vi "Init Robot - Copy.vi"(8 "Brake Switch 35":bool=TRUE, 9 "Brake Switch 40":bool=TRUE, 10 "Brake 40":bool=TRUE, 11 "Brake 35":bool=TRUE) -> (0 "Force bias PS_R":dbl, 1 "Force bias GR_R":dbl, 2 "Potentiometers Diff Too Much":bool, 3 "Init values":dbl[](array[numeric]), 4 "Force Sensor Faulty":bool, 5 "Bias PS_L":dbl, 7 "Bias GR_L":dbl)   [LabVIEW 2019]
uses:
  <vilib>/myRIO/Common/Instrument Driver Framework/myRIO v1.0/Encoder/typedefs/Encoder Count Direction Enum.ctl
  <vilib>/myRIO/Common/Instrument Driver Framework/myRIO v1.0/Encoder/typedefs/Encoder Signal Mode.ctl
  <vilib>/myRIO/Common/Instrument Driver Framework/myRIO v1.0/Encoder/typedefs/Encoder Channels Enum.ctl
  <vilib>/myRIO/Common/Instrument Driver Framework/Utilities/typedefs/Generic FPGA Reference.ctl
  <vilib>/myRIO/Common/Instrument Driver Framework/Utilities/typedefs/myRIO v1.0 Reference.ctl
  <vilib>/myRIO/Common/Instrument Driver Framework/Utilities/typedefs/Hardware Version Enum.ctl
  <vilib>/myRIO/Common/Instrument Driver Framework/Utilities/typedefs/myRIO Generic Hardware Reference.ctl
  <vilib>/myRIO/Instrument Drivers/Onboard IO/Encoder/typedefs/Encoder Reference.ctl
  <vilib>/myRIO/Instrument Drivers/Onboard IO/Encoder/Encoder.lvlib
  <vilib>/myRIO/Instrument Drivers/Onboard IO/Encoder/vis/Read.vi
  <vilib>/myRIO/Common/Instrument Driver Framework/myRIO v1.0/Encoder/typedefs/Encoder Configuration v1.0.ctl
  <vilib>/userDefined/High Color/nirio_resource_hc.ctl
  <vilib>/myRIO/Common/Instrument Driver Framework/myRIO v1.0/Encoder/vis/myRIO v1.0 Configure Encoder.vi
  <vilib>/myRIO/Instrument Drivers/Onboard IO/Encoder/vis/myRIO Encoder Open.xnode
  <vilib>/myRIO/Common/Instrument Driver Framework/Utilities/vis/Is FPGA Ref Available.vi
  <vilib>/myRIO/Express VI/Onboard IO/Encoder/Encoder Express VI.xnode
  <vilib>/myRIO/Express VI/Onboard IO/DO/DO Express VI.xnode
  <vilib>/myRIO/Instrument Drivers/Onboard IO/DIO/vis/Write.vi
  <vilib>/myRIO/Instrument Drivers/Onboard IO/DIO/DIO.lvlib
  <vilib>/myRIO/Common/Instrument Driver Framework/myRIO v1.0/DIO/typedefs/DIO Channels Enum.ctl
  <vilib>/myRIO/Common/Instrument Driver Framework/myRIO v1.0/DIO/typedefs/DIO Channels List.ctl
  <vilib>/myRIO/Instrument Drivers/Onboard IO/DIO/typedefs/DIO Reference.ctl
  <vilib>/myRIO/Instrument Drivers/Onboard IO/DIO/vis/myRIO DIO Open.xnode
  <vilib>/myRIO/Express VI/Onboard IO/AI/AI Express VI.xnode
  <vilib>/myRIO/Common/Instrument Driver Framework/Utilities/typedefs/Analog Scaling Constants.ctl
  <vilib>/myRIO/Common/Instrument Driver Framework/Utilities/typedefs/Analog Scaling Constants List.ctl
  <vilib>/myRIO/Common/Instrument Driver Framework/myRIO v1.0/AO/typedefs/AO Channels Enum.ctl
  <vilib>/myRIO/Common/Instrument Driver Framework/myRIO v1.0/AO/typedefs/AO Channels List.ctl
  <vilib>/myRIO/Instrument Drivers/Onboard IO/AO/typedefs/AO Reference.ctl
  <vilib>/myRIO/Instrument Drivers/Onboard IO/AO/AO.lvlib
  <vilib>/myRIO/Instrument Drivers/Onboard IO/AO/vis/Write.vi
  <vilib>/myRIO/Instrument Drivers/Onboard IO/AO/vis/myRIO AO Open.xnode
  <vilib>/myRIO/Express VI/Onboard IO/AO/AO Express VI.xnode
  <vilib>/myRIO/Instrument Drivers/Onboard IO/AI/vis/Read.vi
  <vilib>/myRIO/Instrument Drivers/Onboard IO/AI/AI.lvlib
  <vilib>/myRIO/Common/Instrument Driver Framework/myRIO v1.0/AI/typedefs/AI Channels Enum.ctl
  <vilib>/myRIO/Common/Instrument Driver Framework/myRIO v1.0/AI/typedefs/AI Channels List.ctl
  <vilib>/myRIO/Instrument Drivers/Onboard IO/AI/typedefs/AI Reference.ctl
  <vilib>/myRIO/Instrument Drivers/Onboard IO/AI/vis/myRIO AI Open.xnode
  <vilib>/myRIO/Common/Instrument Driver Framework/myRIO v1.0/DIO/vis/myRIO v1.1 Open DIO.vi
  <vilib>/myRIO/Common/Instrument Driver Framework/myRIO v1.0/AI/vis/myRIO v1.1 Open AI.vi
  <vilib>/myRIO/Common/Instrument Driver Framework/myRIO v1.0/Encoder/vis/myRIO v1.1 Open Encoder.vi
  <vilib>/myRIO/Common/Instrument Driver Framework/myRIO v1.0/AO/vis/myRIO v1.1 Open AO.vi
panel:
  out "Init Values":dbl[](array[numeric])
  out "Bias GR_R":dbl
  out "Bias PS_R":dbl
  out "VoltageTranslation":dbl
  out "VoltageRotation":dbl
  out "Force bias PS_L":dbl
  out "Force bias GR_L":dbl
  out "Encoder Counter Value":i32(graph)
  out "Encoder Counter Value 2":i32(graph)
  out "Volt L":dbl
  out "Rot Volt":dbl
  out "Volt R":dbl
  out "E rotation":dbl
  out "E translation":dbl
  out "P Rotation":dbl
  out "P Translation":dbl
  out "left init":dbl
  out "right init":dbl
  out "SCAIME":dbl
  # "This Vi starts all task, calculates the initals values of all sensores and encoder and can open the brakes if needed."
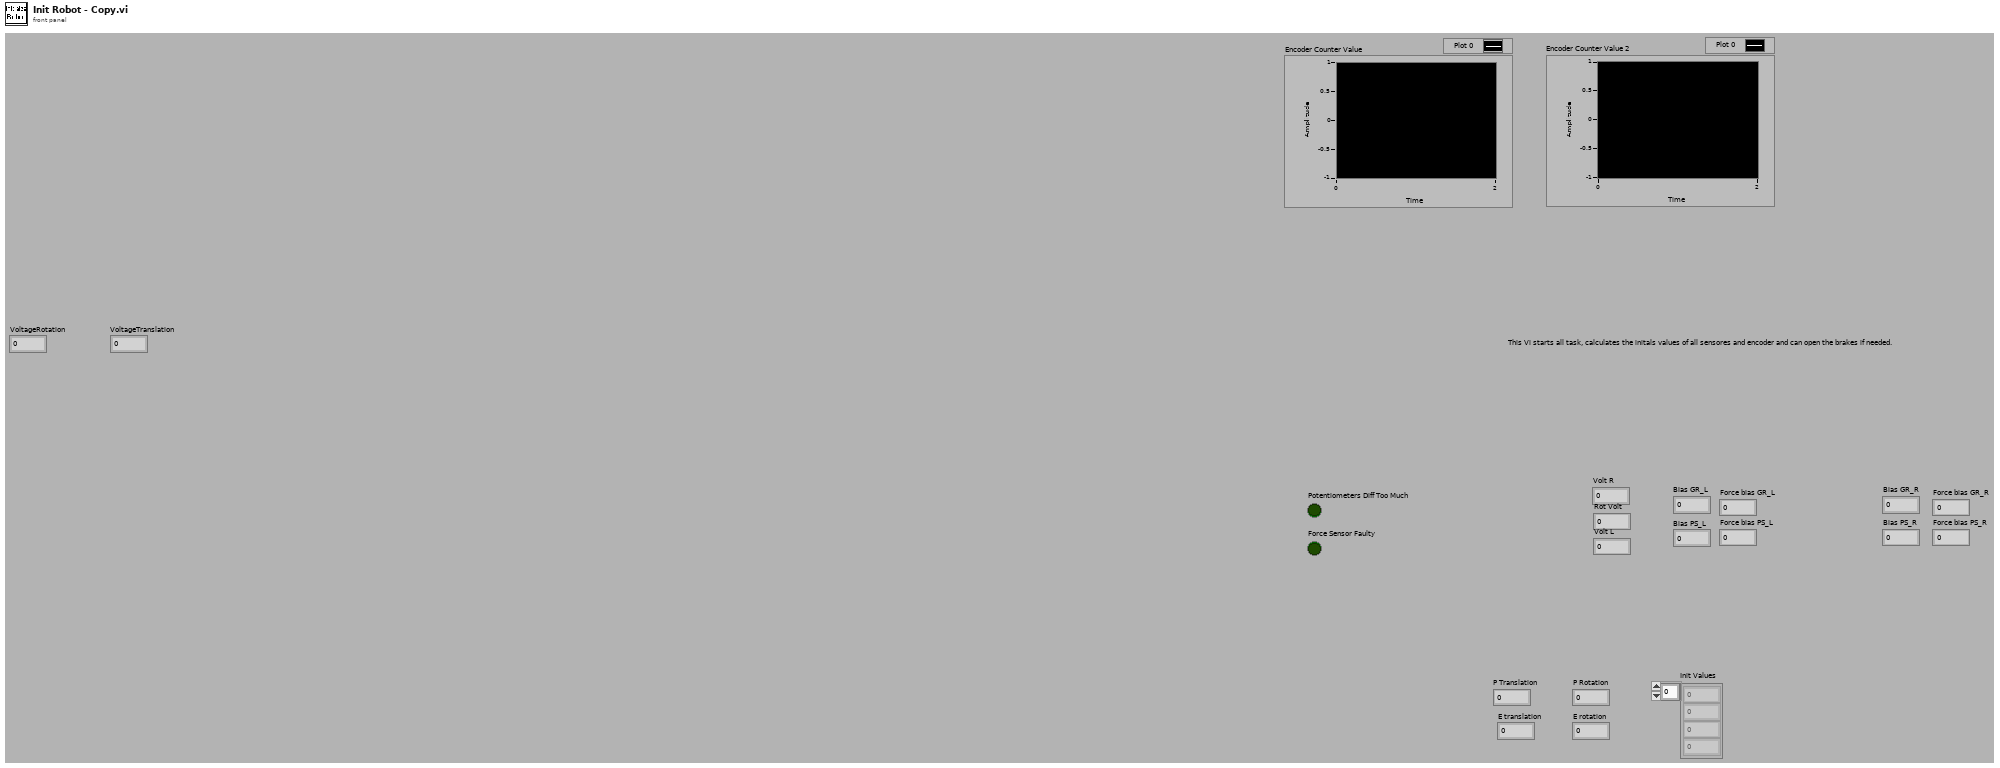
[diagram p1: front panel]
types:
  T1 = typedef "AO.lvlib/AO Reference.ctl" = cluster{"myRIO Reference":T2, "AO Channel List":T6, "AO Scaling Constant List":T8}
  T2 = typedef "myRIO Generic Hardware Reference.ctl" = cluster{"myRIO Model":T3, "myRIO Hardware Reference":T4}
  T3 = typedef "Hardware Version Enum.ctl" = enum16{"Unknown", "myRIO-1900", "myRIO-1950", "roboRIO", "NI ELVIS RIO CM", "ELVIS III"}
  T4 = typedef "myRIO v1.0 Reference.ctl" = cluster{"Generic FPGA Reference":T5, "Allow multiple opens":bool}
  T5 = typedef "Generic FPGA Reference.ctl" = refnum<k20>
  T6 = typedef "AO Channels List.ctl" = T7[]
  T7 = typedef "AO Channels Enum.ctl" = enum16{"Not Connected", "AudioOut/Left", "AudioOut/Right", "C/AO0", "C/AO1", "A/AO0", "A/AO1", "B/AO0", "B/AO1"}
  T8 = typedef "Analog Scaling Constants List.ctl" = T9[]
  T9 = typedef "Analog Scaling Constants.ctl" = cluster{"LSB Weight (Volts)":dbl, "Offset (Volts)":dbl, "Signed?":bool}
  T10 = typedef "nirio_resource_hc.ctl" = tag
  T11 = typedef "DIO.lvlib/DIO Reference.ctl" = cluster{"myRIO Reference":T2, "DIO Channels List":T12}
  T12 = typedef "DIO Channels List.ctl" = T13[]
  T13 = typedef "DIO Channels Enum.ctl" = enum16{"Not Connected", "C/DIO0", "C/DIO1", "C/DIO2", "C/DIO3", "C/DIO4", "C/DIO5", "C/DIO6", "C/DIO7", "A/DIO0", "A/DIO1", "A/DIO2", "A/DIO3", "A/DIO4", "A/DIO5", "A/DIO6", "A/DIO7", "A/DIO8", "A/DIO9", "A/DIO10", "A/DIO11", "A/DIO12", "A/DIO13", "A/DIO14", "A/DIO15", "A/DIO16", "A/DIO17", "A/DIO18", "A/DIO19", "B/DIO0", "B/DIO1", "B/DIO2", "B/DIO3", "B/DIO4", "B/DIO5", "B/DIO6", "B/DIO7", "B/DIO8", "B/DIO9", "B/DIO10", "B/DIO11", "B/DIO12", "B/DIO13", "B/DIO14", "B/DIO15", "B/DIO16", "B/DIO17", "B/DIO18", "B/DIO19", "LED0", "LED1", "LED2", "LED3", "Button0", "DIO/DIO0", "DIO/DIO1", "DIO/DIO2", "DIO/DIO3", "DIO/DIO4", "DIO/DIO5", "DIO/DIO6", "DIO/DIO7", "DIO/DIO8", "DIO/DIO9", "SPI/CS0", "SPI/CS1", "SPI/CS2", "SPI/CS3", "LED RADIO (Green)", "LED RADIO (Red)", "LED COMM (Green)", "LED COMM (Red)", "LED MODE (Green)", "LED MODE (Red)"}
  T14 = typedef "AI.lvlib/AI Reference.ctl" = cluster{"myRIO Reference":T2, "AI Channels List":T15, "AI Scaling Constants List":T8}
  T15 = typedef "AI Channels List.ctl" = T16[]
  T16 = typedef "AI Channels Enum.ctl" = enum16{"Not Connected", "AudioIn/Left", "AudioIn/Right", "C/AI0", "C/AI1", "A/AI0", "A/AI1", "A/AI2", "A/AI3", "A/AI4", "A/AI5", "A/AI6", "A/AI7", "B/AI0", "B/AI1", "B/AI2", "B/AI3", "B/AI4", "B/AI5", "B/AI6", "B/AI7", "AI/AI0", "AI/AI1", "AI/AI2", "AI/AI3", "A/AI0 (DIFF)", "A/AI1 (DIFF)", "A/AI2 (DIFF)", "A/AI3 (DIFF)", "B/AI0 (DIFF)", "B/AI1 (DIFF)", "B/AI2 (DIFF)", "B/AI3 (DIFF)"}
  T17 = typedef "Encoder.lvlib/Encoder Reference.ctl" = cluster{"myRIO Reference":T2, "Encoder Channels Enum":T18}
  T18 = typedef "Encoder Channels Enum.ctl" = enum16{"Not Connected", "C/ENC0", "C/ENC1", "A/ENC", "A/ENC0", "A/ENC1", "A/ENC2", "A/ENC3", "A/ENC4", "A/ENC5", "A/ENC6", "A/ENC7", "A/ENC8", "A/ENC9", "B/ENC", "B/ENC0", "B/ENC1", "B/ENC2", "B/ENC3", "B/ENC4", "B/ENC5", "B/ENC6", "B/ENC7", "B/ENC8", "B/ENC9", "DIO/ENC0", "DIO/ENC1", "DIO/ENC2", "DIO/ENC3", "DIO/ENC4"}
  T19 = typedef "Encoder Signal Mode.ctl" = enum16{"Quadrature phase signal", "Step and direction signal"}
  T20 = cluster{"[0]":dbl, "[1]":dbl, "[2]":dbl, "[3]":dbl, "[4]":dbl, "[5]":dbl, "[6]":dbl, "[7]":dbl, "[8]":dbl}
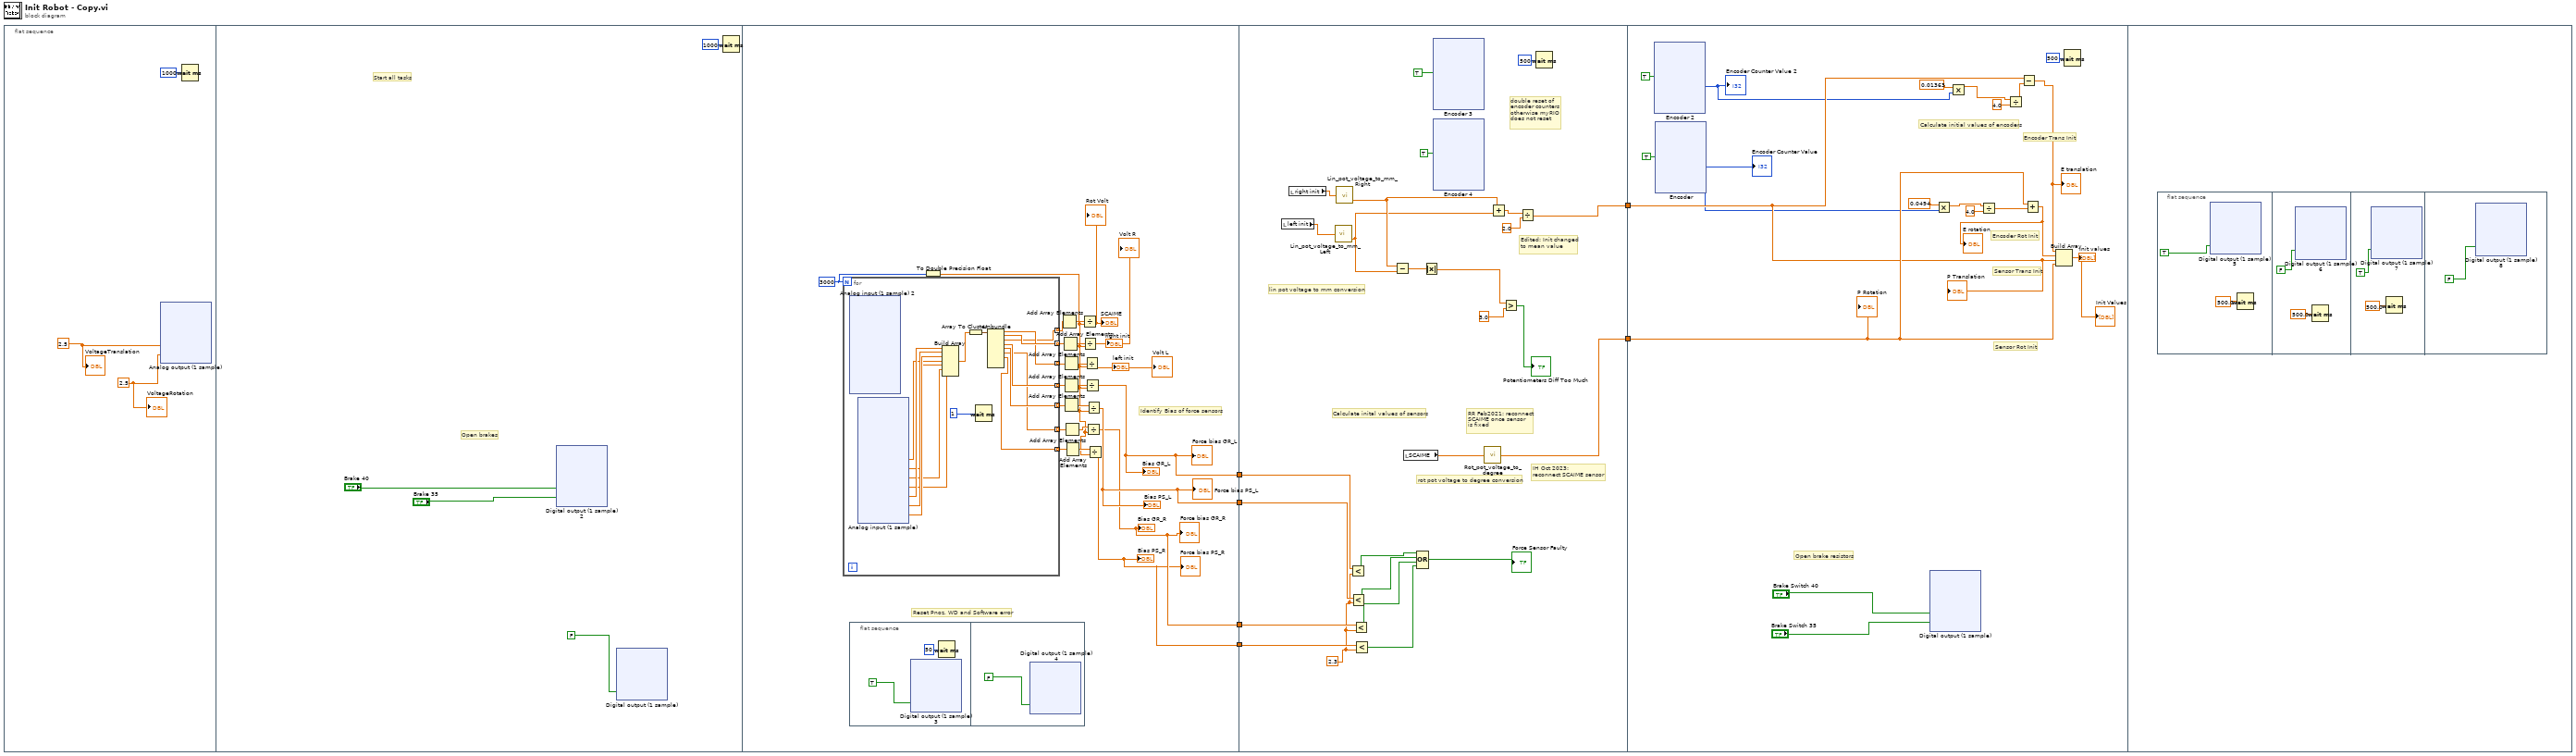
[diagram p0: block diagram]
diagram:
  n1 = flat-sequence {
    tunnel: [w126] -> w4
    tunnel: [w125] -> w3
    tunnel: [w124] -> w2
    tunnel: [w123] -> w1
    tunnel: [w337] -> w6
    tunnel: [w320] -> w5
    tunnel: w4 -> [w329]
    tunnel: w3 -> [w328]
    tunnel: w2 -> [w327]
    tunnel: w1 -> [w326]
    tunnel: w6 -> [w452]
    tunnel: w5 -> [w453]
    frame #0 {
      w7 = 2.5
      w8 = 2.5
      n2 = xnode "Analog output (1 sample)"("Motor1Current_AREAD (B/AO0 (Pin 2))"=w8, "Motor2Current_AREAD (A/AO0 (Pin 2))"=w7) -> ()  [unwired: 1 in, 1 out]
      n3 = Wait (ms)(milliseconds to wait=u32 1000) -> ()  [unwired: 1 out]
      "VoltageRotation" <- w7
      "VoltageTranslation" <- w8
    }
    frame #1 {
      # "Open brakes"
      # "Start all tasks"
      n4 = xnode "Digital output (1 sample) 2"("SIG_REL3 (B/DIO2 (Pin 15))"="Brake 40", "SIG_REL5 (B/DIO4 (Pin 19))"="Brake 35") -> ()  [unwired: 1 in, 1 out]
      n5 = xnode "Digital output (1 sample)"("Safety PILZ (B/DIO0 (Pin 11))"=FALSE ("data")) -> ()  [unwired: 1 in, 1 out]
      n6 = Wait (ms)(milliseconds to wait=u32 1000) -> ()  [unwired: 1 out]
    }
    frame #2 {
      w137 = 3000
      # "Identify Bias of force sensors"
      # "Reset Pnoz, WD and Software error"
      n7 = for {
        N: w137 -> [_]
        tunnel: [w155] -> w142 mode=indexing
        tunnel: [w161] -> w141 mode=indexing
        tunnel: [w156] -> w140 mode=indexing
        tunnel: [w158] -> w133 mode=indexing
        tunnel: [w157] -> w132 mode=indexing
        tunnel: [w151] -> w128 mode=indexing
        tunnel: [w150] -> w127 mode=indexing
        n8 = xnode "Analog input (1 sample) 2"() -> ()  [unwired: 1 in, 6 out]
        n9 = xnode "Analog input (1 sample)"() -> ("ForceSensor_READ1 (C/AI0 (AI0))"=w147:dbl, "ForceSensor_READ2 (C/AI1 (AI1))"=w146:dbl, "ForceSensor_READ3 (B/AI0 (Pin 3))"=w149:dbl, "ForceSensor_READ4 (B/AI1 (Pin 5))"=w148:dbl, "AI_lin_pot_left (A/AI0 (Pin 3))"=w154:dbl, "AI_lin_pot_right (A/AI1 (Pin 5))"=w153:dbl, "AI_rot_pot (A/AI2 (Pin 7))"=w152:dbl)  [unwired: 1 in, 1 out]
        n10 = Build Array(w154, w153, w152, w147, w146, w149, w148) -> (w159:dbl[])
        n11 = Array To Cluster(array=w159) -> (cluster=w162:T20)
        n12 = Wait (ms)(milliseconds to wait=1) -> ()  [unwired: 1 out]
        n13 = Unbundle(w162) -> ("[0]"=w156:dbl, "[1]"=w161:dbl, "[2]"=w155:dbl, "[3]"=w158:dbl, "[4]"=w157:dbl, "[5]"=w151:dbl, "[6]"=w150:dbl)  [unwired: 2 out]
      }
      n14 = flat-sequence {
        frame #0 {
          n15 = xnode "Digital output (1 sample) 3"("Safety PILZ (B/DIO0 (Pin 11))"=TRUE ("data")) -> ()  [unwired: 1 in, 1 out]
          n16 = Wait (ms)(milliseconds to wait=u32 50) -> ()  [unwired: 1 out]
        }
        frame #1 {
          n17 = xnode "Digital output (1 sample) 4"("Safety PILZ (B/DIO0 (Pin 11))"=FALSE ("data")) -> ()  [unwired: 1 in, 1 out]
        }
      }
      n18 = To Double Precision Float(number=w137) -> (double precision float=w129:dbl)
      n19 = Add Array Elements(numeric array=w142) -> (sum=w145:dbl)
      n20 = Add Array Elements(numeric array=w141) -> (sum=w144:dbl)
      n21 = Add Array Elements(numeric array=w133) -> (sum=w135:dbl)
      n22 = Add Array Elements(numeric array=w140) -> (sum=w143:dbl)
      n23 = Add Array Elements(numeric array=w132) -> (sum=w134:dbl)
      n24 = Add Array Elements(numeric array=w128) -> (sum=w130:dbl)
      n25 = Add Array Elements(numeric array=w127) -> (sum=w131:dbl)
      n26 = Divide(x=w145, y=w129) -> (x/y=→"SCAIME" →"Rot Volt":dbl)
      n27 = Divide(x=w144, y=w129) -> (x/y=→"right init" →"Volt R":dbl)
      n28 = Divide(x=w143, y=w129) -> (x/y=→"left init" →"Volt L":dbl)
      n29 = Divide(x=w135, y=w129) -> (x/y=w126:dbl)
      "Force bias GR_L" <- w126
      "Bias GR_L" <- w126
      n30 = Divide(x=w130, y=w129) -> (x/y=w124:dbl)
      "Bias GR_R" <- w124
      "Force bias GR_R" <- w124
      n31 = Divide(x=w134, y=w129) -> (x/y=w125:dbl)
      "Force bias PS_L" <- w125
      "Bias PS_L" <- w125
      n32 = Divide(x=w131, y=w129) -> (x/y=w123:dbl)
      "Bias PS_R" <- w123
      "Force bias PS_R" <- w123
    }
    frame #3 {
      w325 = 2.3
      # "IH Oct 2023: \nreconnect SCAIME sensor"
      # "Edited: Init changed to mean value"
      # "lin pot voltage to mm conversion"
      # "rot pot voltage to degree conversion"
      # "RR Feb2021: reconnect\nSCAIME once sensor\nis fixed"
      # "double reset of\nencoder counters\notherwise myRIO\ndoes not reset"
      # "Calculate inital values of sensors"
      n33 = local read "left init"() -> (w340:dbl)
      n34 = local read "right init"() -> (w341:dbl)
      n35 = call "Lin_pot_voltage_to_mm_Left.vi"("LinPot Voltage"=w340) -> ("LinPot mm (center to finger)"=w335:dbl)  [unwired: 1 out]
      n36 = call "Lin_pot_voltage_to_mm_Right.vi"("LinPot Voltage"=w341) -> ("LinPot mm (center to finger)"=w336:dbl)  [unwired: 1 out]
      n37 = Less?(x=w329, y=w325) -> (x < y?=w324:bool)
      n38 = Less?(x=w328, y=w325) -> (x < y?=w323:bool)
      n39 = Less?(x=w327, y=w325) -> (x < y?=w322:bool)
      n40 = Less?(x=w326, y=w325) -> (x < y?=w321:bool)
      n41 = Subtract(x=w336, y=w335) -> (x-y=w332:dbl)
      n42 = local read "SCAIME"() -> (w342:dbl)
      n43 = Compound Arithmetic op=OR(w324, w323, w322, w321) -> (→"Force Sensor Faulty":bool)
      n44 = Absolute Value(x=w332) -> (abs(x)=w331:dbl)
      n45 = xnode "Encoder 3"("Reset Counter"=TRUE) -> ()  [unwired: 1 in, 4 out]
      n46 = xnode "Encoder 4"("Reset Counter"=TRUE) -> ()  [unwired: 1 in, 4 out]
      n47 = call "Rot_pot_voltage_to_degree.vi"("RotaryPot (Voltage)"=w342) -> ("RotaryPot (degree)"=w320:dbl)
      n48 = Add(x=w336, y=w335) -> (x+y=w339:dbl)
      n49 = Greater?(x=w331, y=3.0) -> (0:→"Potentiometers Diff Too Much":bool)
      n50 = Divide(x=w339, y=2.0) -> (x/y=w337:dbl)
      n51 = Wait (ms)(milliseconds to wait=u32 500) -> ()  [unwired: 1 out]
    }
    frame #4 {
      # "Calculate initial values of encoders"
      # "Open brake resistors"
      # "Encoder Trans Init"
      # "Encoder Rot Init"
      # "Sensor Trans Init"
      # "Sensor Rot Init"
      n52 = xnode "Encoder 2"("Reset Counter"=TRUE) -> ("Counter Value"=w451:i32)  [unwired: 1 in, 3 out]
      "Encoder Counter Value 2" <- w451
      n53 = xnode "Encoder"("Reset Counter"=TRUE) -> ("Counter Value"=w450:i32)  [unwired: 1 in, 3 out]
      "Encoder Counter Value" <- w450
      n54 = xnode "Digital output (1 sample)"("SIG_REL2 (B/DIO1 (Pin 13))"="Brake Switch 40", "SIG_REL4 (B/DIO3 (Pin 17))"="Brake Switch 35") -> ()  [unwired: 1 in, 1 out]
      n55 = Multiply(x=0.0494, y=w450) -> (x*y=w443:dbl)
      n56 = Multiply(x=0.01363, y=w451) -> (x*y=w440:dbl)
      n57 = Divide(x=w443, y=4.0) -> (x/y=w442:dbl)
      n58 = Divide(x=w440, y=4.0) -> (x/y=w439:dbl)
      n59 = Subtract(x=w452, y=w439) -> (x-y=w441:dbl)
      "E translation" <- w441
      n60 = Add(x=w453, y=w442) -> (x+y=w454:dbl)
      "E rotation" <- w454
      n61 = Build Array(w441, w454, w452, w453) -> (→"Init values" →"Init Values":dbl[])
      n62 = Wait (ms)(milliseconds to wait=u32 500) -> ()  [unwired: 1 out]
      "P Translation" <- w452
      "P Rotation" <- w453
    }
    frame #5 {
      n63 = flat-sequence {
        frame #0 {
          n64 = xnode "Digital output (1 sample) 5"("C/DIO7 (DIO7)"=TRUE) -> ()  [unwired: 1 in, 1 out]
          n65 = Wait (ms)(milliseconds to wait=500.0) -> ()  [unwired: 1 out]
        }
        frame #1 {
          n66 = xnode "Digital output (1 sample) 6"("C/DIO7 (DIO7)"=FALSE) -> ()  [unwired: 1 in, 1 out]
          n67 = Wait (ms)(milliseconds to wait=500.0) -> ()  [unwired: 1 out]
        }
        frame #2 {
          n68 = xnode "Digital output (1 sample) 7"("C/DIO7 (DIO7)"=TRUE) -> ()  [unwired: 1 in, 1 out]
          n69 = Wait (ms)(milliseconds to wait=500.0) -> ()  [unwired: 1 out]
        }
        frame #3 {
          n70 = xnode "Digital output (1 sample) 8"("C/DIO7 (DIO7)"=FALSE) -> ()  [unwired: 1 in, 1 out]
        }
      }
    }
  }
